vi "Initialize Lookup Table - Ramp.vi"() -> ()   [LabVIEW 2015]
uses:
  <vilib>/Analysis/1siggen.llb/Ramp Pattern by Samples.vi
  <vilib>/Analysis/NI_AALBase.lvlib
panel:
  in  "flyback":ext=0.2
  out "波形图":i16[](graph)
  out "Init Data Out":i16[](array[numeric])
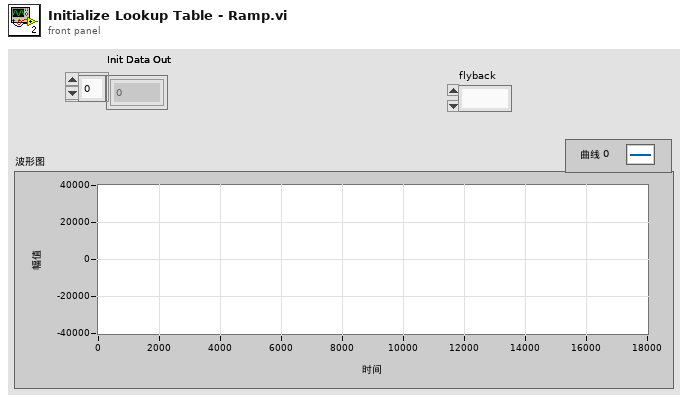
[diagram p1: front panel]
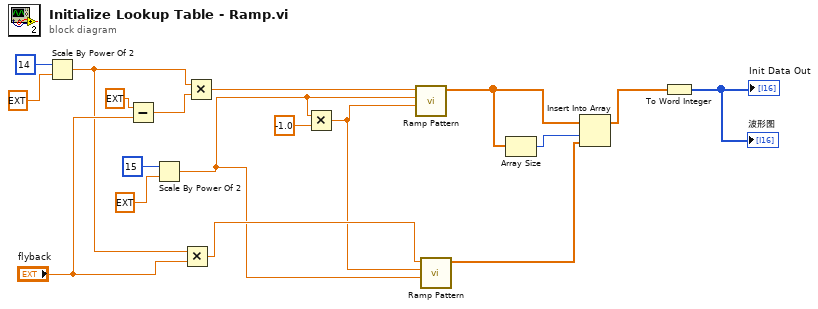
[diagram p0: block diagram]
diagram:
  n1 = Scale By Power Of 2(n=i16 14, x=ext 1.0) -> (x*2^n=w3:ext)
  n2 = Subtract(x=ext 1.0, y="flyback") -> (x-y=w6:ext)
  n3 = Scale By Power Of 2(n=i16 15, x=ext 1.0) -> (x*2^n=w1:ext)
  n4 = Multiply(x=w3, y="flyback") -> (x*y=w13:ext)
  n5 = Multiply(x=w3, y=w6) -> (x*y=w14:ext)
  n6 = Multiply(x=w1, y=-1.0) -> (x*y=w2:ext)
  n7 = call-poly <vilib>:"Ramp Pattern.vi"("start"=w2, "end"=w1, "samples"=w14) -> ("Ramp Pattern"=w11:dbl[])  [unwired: 7 in, 1 out]
  n8 = call-poly <vilib>:"Ramp Pattern.vi"("start"=w1, "end"=w2, "samples"=w13) -> ("Ramp Pattern"=w10:dbl[])  [unwired: 7 in, 1 out]
  n9 = Array Size(array=w11) -> (size(s)=w8:i32)
  n10 = Insert Into Array(array=w11, index=w8, new element=w10) -> (w12:dbl[])
  n11 = To Word Integer(number=w12) -> (16bit integer=→"Init Data Out" →"波形图":i16[])
